vi "ESR.vi"(8 "error in (no error)":errorcluster, 10 "Node In":string, 11 "VISA resource name":refnum<visa-resource-name>) -> (0 "error out":errorcluster, 1 "ESR":u8, 2 "Node Out":string, 3 "VISA resource name out":refnum<visa-resource-name>, 4 "Command String":string)   [LabVIEW 2013, in "Keithley 2600 Series.lvlib"]
doc: "Standard Event Status Register query. *ESR?\n\n<b>Functions and Attributes Used</b>\nstatus.standard.event"
uses:
  Keithley 2600 Series.lvlib
panel:
  # "(c) 2008 Keithley Instruments, Inc.  ALL RIGHTS RESERVED."
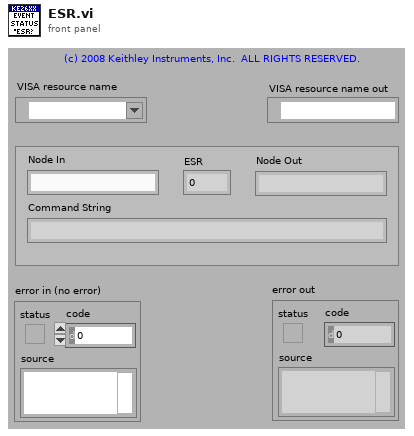
[diagram p1: front panel]
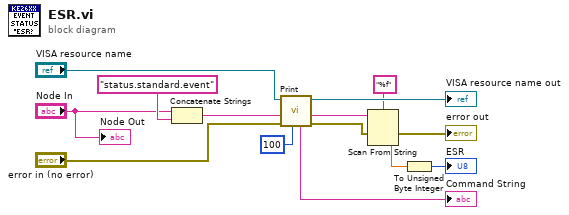
[diagram p0: block diagram]
diagram:
  n1 = Concatenate Strings("Node In", "status.standard.event" ("string")) -> (w12:string)
  n2 = call "Print.vi"("Byte Count (1024)"=u32 100, "error in (no error)"="error in (no error)", "Input"=w12, "VISA resource name"="VISA resource name") -> ("error out"=w4:errorcluster, "Output"=w6:string, "VISA resource name out"=→"VISA resource name out":refnum<visa-resource-name>, "Command String"=→"Command String":string)  [unwired: 1 in, 3 out]
  n3 = Scan From String(format string="%f", input string=w6, error in=w4) -> (error out=→"error out":errorcluster, output 1=w2:dbl)  [unwired: 1 in, 3 out]
  n4 = To Unsigned Byte Integer(number=w2) -> (unsigned 8bit integer=→"ESR":u8)
  "Node Out" <- "Node In"
